vi "Untitled 1.vi"() -> ()   [LabVIEW 2015]
uses:
  Control 1.ctl
panel:
  in  "Take food":bool
  out "Screen":bool
  out "2D Picture":picture
  in  "Enum":T1
  in  "Open":bool
  in  "Power":u8(knob) scale=0.0..10.0
  in  "Time":u8(knob) scale=0.0..30.0
  in  "stop":bool
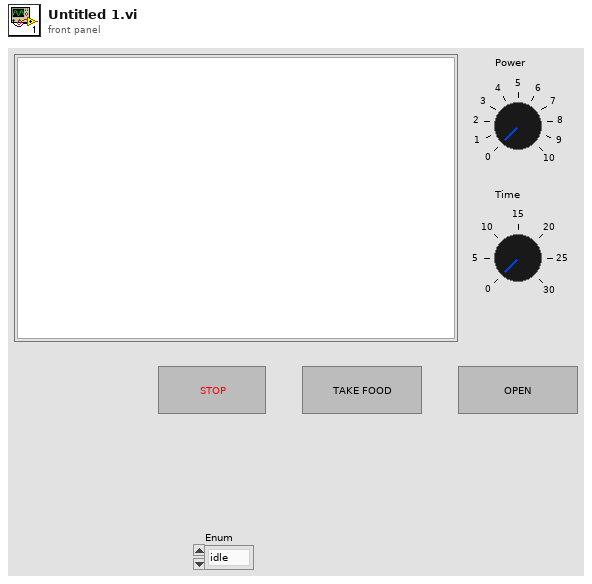
[diagram p1: front panel]
types:
  T1 = typedef "Control 1.ctl" = enum16{"idle ", "opened", "working", "done", "end", ""}
  T2 = typedef "imagedata.ctl" = cluster{"image type":i32, "image depth":i32, "image":u8[], "mask":u8[], "colors":u32[], "Rectangle":cluster{"left":i16, "top":i16, "right":i16, "bottom":i16}}
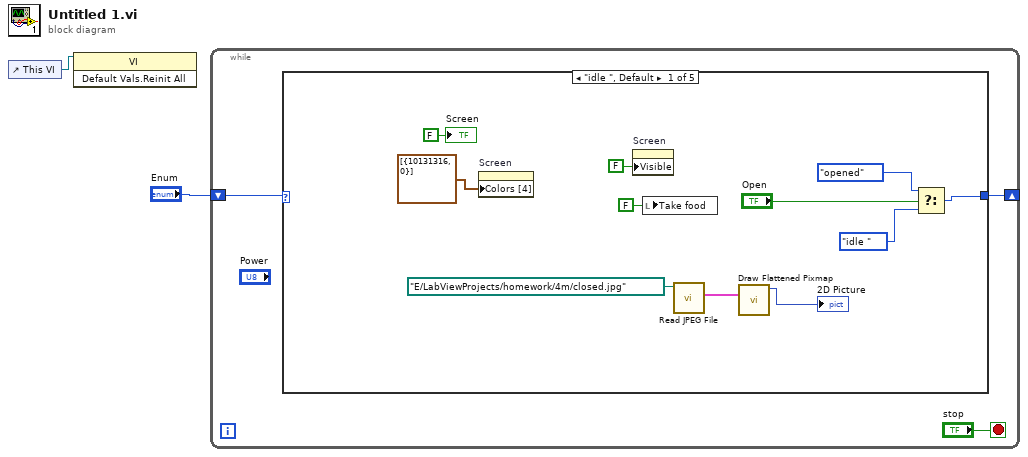
[diagram p0: block diagram]
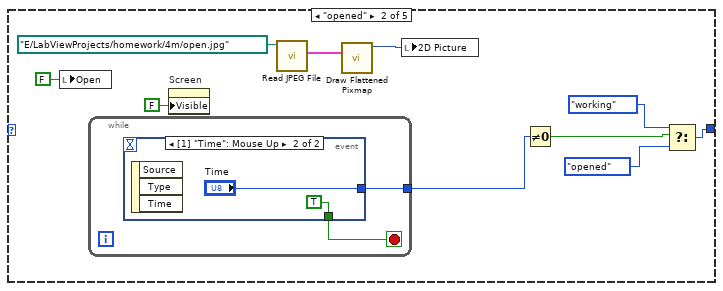
[diagram p2: hidden frame]
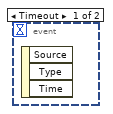
[diagram p3: hidden frame]
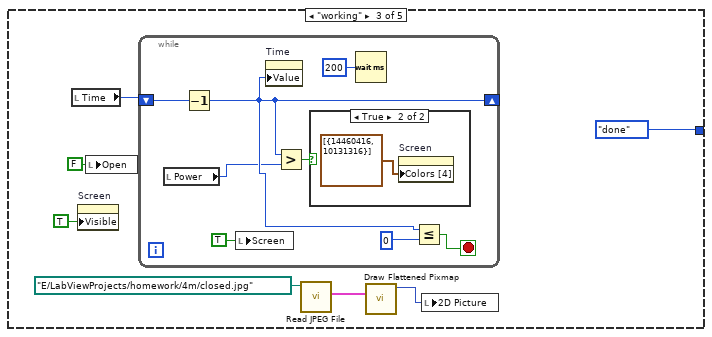
[diagram p4: hidden frame]
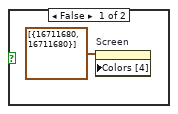
[diagram p5: hidden frame]
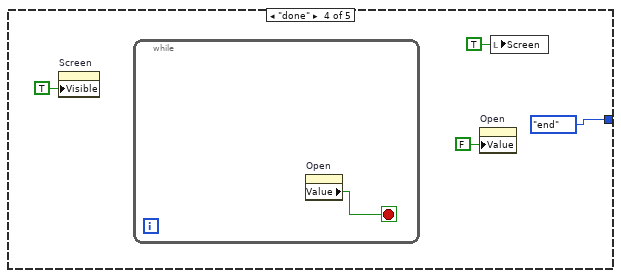
[diagram p6: hidden frame]
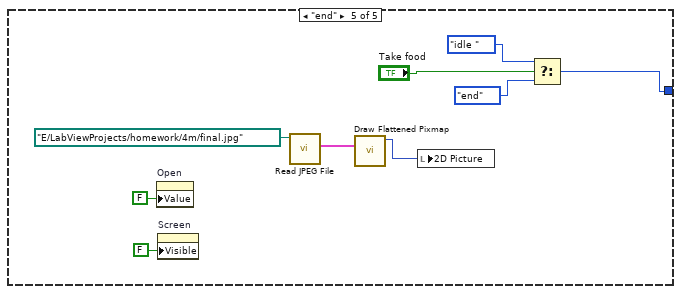
[diagram p7: hidden frame]
diagram:
  n1 = control-ref of="This VI"() -> (w2:refnum<vi>)
  n2 = invoke class="VI" method="Default Vals.Reinit All"(reference=w2) -> ()  [unwired: 2 in, 3 out]
  n3 = while {
    shift-right: [w4] -> _
    shift-left: "Enum" -> [w3]
    stop <- "stop" stop-if-true
    n4 = case shown="\"idle \", Default" w3 {
      tunnel: [w14 w25 Control_1."done" ("Enum") Control_1."end" ("Enum") w56] -> w4
      frame "idle ", Default {
        n5 = property on="Screen" class="Bool (strict)"("Colors [4]"=cluster{u32, u32}[] [{10131316, 0}]) -> ()  [unwired: 2 in, 2 out]
        n6 = property on="Screen" class="Bool (strict)"("Visible"=FALSE) -> ()  [unwired: 2 in, 2 out]
        n7 = local write "Take food"(FALSE ("Take food")) -> ()
        n8 = call <vilib>:"Read JPEG File.vi"("path to JPEG file"=path "E:/LabViewProjects/homework/4m/closed.jpg") -> ("image data"=w11:T2)  [unwired: 8 in, 2 out]
        n9 = call <vilib>:"Draw Flattened Pixmap.vi"("image data"=w11) -> ("new picture"=→"2D Picture":picture)  [unwired: 8 in]
        n10 = Select(t=Control_1."opened" ("Enum"), s="Open", f=Control_1."idle " ("Enum")) -> (s? t:f=w14:T1)
        "Screen" <- FALSE ("Screen")
      }
      frame "opened" {
        n11 = local write "Open"(FALSE ("Open")) -> ()
        n12 = while {
          tunnel: [w28] -> w20
          stop <- w27 stop-if-true
          n13 = event shown="[1] \"Time\": Mouse Up" {
            selector: _ -> [_ _]
            dyn-events: _ -> [_ _]
            timeout: _ -> [_ _]
            tunnel: [_ "Time"] -> w28
            tunnel: [_ TRUE] -> w27
            event Timeout {
              n14 = event-data() -> ()  [unwired: 1 in, 3 out]
            }
            event "Time": Mouse Up {
              n15 = event-data() -> ()  [unwired: 1 in, 3 out]
            }
          }
        }
        n16 = property on="Screen" class="Bool (strict)"("Visible"=FALSE) -> ()  [unwired: 2 in, 2 out]
        n17 = call <vilib>:"Read JPEG File.vi"("path to JPEG file"=path "E:/LabViewProjects/homework/4m/open.jpg") -> ("image data"=w26:T2)  [unwired: 8 in, 2 out]
        n18 = call <vilib>:"Draw Flattened Pixmap.vi"("image data"=w26) -> ("new picture"=w23:picture)  [unwired: 8 in]
        n19 = local write "2D Picture"(w23) -> ()
        n20 = Not Equal To 0?(x=w20) -> (x != 0?=w21:bool)
        n21 = Select(t=Control_1."working" ("Enum"), s=w21, f=Control_1."opened" ("Enum")) -> (s? t:f=w25:T1)
      }
      frame "working" {
        n22 = local read "Time"() -> (w36:u8)
        n23 = property on="Screen" class="Bool (strict)"("Visible"=TRUE) -> ()  [unwired: 2 in, 2 out]
        n24 = local write "Open"(FALSE ("Open")) -> ()
        n25 = while {
          shift-right: [w39] -> _
          shift-left: w36 -> [w44]
          stop <- w41 stop-if-true
          n26 = local read "Power"() -> (w38:u8)
          n27 = Decrement(x=w44) -> (x-1=w39:u8)
          n28 = local write "Screen"(TRUE ("Screen")) -> ()
          n29 = property on="Time" class="Knob (strict)"("Value"=w39) -> ()  [unwired: 2 in, 2 out]
          n30 = Greater?(x=w39, y=w38) -> (0:w43:bool)
          n31 = case shown="True" w43 {
            frame False {
              n32 = property on="Screen" class="Bool (strict)"("Colors [4]"=cluster{u32, u32}[] [{16711680, 16711680}]) -> ()  [unwired: 2 in, 2 out]
            }
            frame True {
              n33 = property on="Screen" class="Bool (strict)"("Colors [4]"=cluster{u32, u32}[] [{14460416, 10131316}]) -> ()  [unwired: 2 in, 2 out]
            }
          }
          n34 = Wait (ms)(milliseconds to wait=u32 200) -> ()  [unwired: 1 out]
          n35 = Less Or Equal?(x=w39, y=u8 0) -> (x <= y?=w41:bool)
        }
        n36 = call <vilib>:"Read JPEG File.vi"("path to JPEG file"=path "E:/LabViewProjects/homework/4m/closed.jpg") -> ("image data"=w33:T2)  [unwired: 8 in, 2 out]
        n37 = call <vilib>:"Draw Flattened Pixmap.vi"("image data"=w33) -> ("new picture"=w34:picture)  [unwired: 8 in]
        n38 = local write "2D Picture"(w34) -> ()
      }
      frame "done" {
        n39 = property on="Screen" class="Bool (strict)"("Visible"=TRUE) -> ()  [unwired: 2 in, 2 out]
        n40 = while {
          stop <- w52 stop-if-true
          n41 = property on="Open" class="Bool (strict)"() -> ("Value"=w52:bool)  [unwired: 2 in, 2 out]
        }
        n42 = property on="Open" class="Bool (strict)"("Value"=FALSE ("Open")) -> ()  [unwired: 2 in, 2 out]
        n43 = local write "Screen"(TRUE ("Screen")) -> ()
      }
      frame "end" {
        n44 = property on="Open" class="Bool (strict)"("Value"=FALSE ("Open")) -> ()  [unwired: 2 in, 2 out]
        n45 = property on="Screen" class="Bool (strict)"("Visible"=FALSE) -> ()  [unwired: 2 in, 2 out]
        n46 = call <vilib>:"Read JPEG File.vi"("path to JPEG file"=path "E:/LabViewProjects/homework/4m/final.jpg") -> ("image data"=w60:T2)  [unwired: 8 in, 2 out]
        n47 = call <vilib>:"Draw Flattened Pixmap.vi"("image data"=w60) -> ("new picture"=w61:picture)  [unwired: 8 in]
        n48 = local write "2D Picture"(w61) -> ()
        n49 = Select(t=Control_1."idle " ("Enum"), s="Take food", f=Control_1."end" ("Enum")) -> (s? t:f=w56:T1)
      }
    }
  }
